vi "TR_Check_files_format.vi"(8 "error in (no error)":errorcluster, 11 "TDMS files paths in":path[](array[path])) -> (0 "error out":errorcluster, 3 "TDMS files paths out":path[](array[path]))   [LabVIEW 2018, in "Tracks Repair.lvlib"]
uses:
  Tracks Repair.lvlib
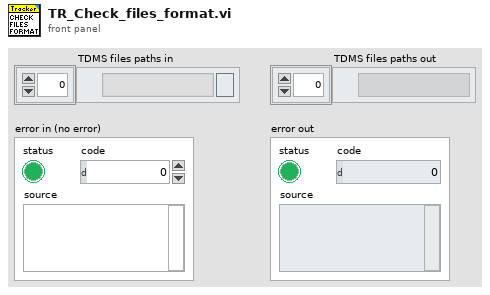
[diagram p1: front panel]
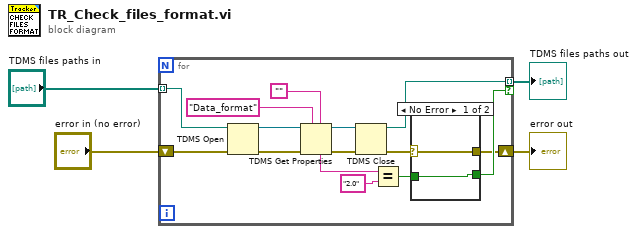
[diagram p0: block diagram]
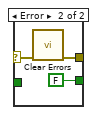
[diagram p2: hidden frame]
diagram:
  n1 = for {
    shift-right: [w5] -> w4
    shift-left: "error in (no error)" -> [w18]
    tunnel: "TDMS files paths in" -> [w19] mode=indexing
    tunnel: [w13] -> w3 mode=indexing if=w7
    n2 = TDMS Open(8:w18, 11:w19) -> (0:w17:errorcluster, 3:w16:refnum<k34>)  [unwired: 5 in]
    n3 = TDMS Get Properties(5:"", 7:"Data_format" ("property name"), 8:w17, 11:w16) -> (0:w14:errorcluster, 3:w15:refnum<k34>, 4:w12:string)  [unwired: 2 in, 3 out]
    n4 = TDMS Close(8:w14, 11:w15) -> (0:w8:errorcluster, 3:w13:path)
    n5 = Equal?(x=w12, y="2.0") -> (x = y?=w6:bool)
    n6 = case shown="No Error" w8 {
      selector: w8 -> [w20 w23]
      tunnel: [w21 FALSE] -> w7
      tunnel: w6 -> [w21 _]
      tunnel: [w20 w22] -> w5
      frame No Error {
      }
      frame Error {
        n7 = call <vilib>:"Clear Errors.vi"("error in (no error)"=w23) -> ("error out"=w22:errorcluster)  [unwired: 5 in, 1 out]
      }
    }
  }
  "error out" <- w4
  "TDMS files paths out" <- w3
